vi "Read.vi"(8 "error in (no error)":errorcluster, 11 "Configuration Filename":path) -> (0 "error out":errorcluster, 1 "All items found?":bool, 2 "HGF_Configuration out":refnum<class "HGF_Configuration.lvclass">, 3 "HGF_Application out":refnum<class "HGF_Application.lvclass">)   [LabVIEW 2012, in "HGF_ApplicationBaseClasses.lvlib" / "HGF_Configuration.lvclass"]
uses:
  HGF_Configuration.lvclass
  HGF_Application/HGF_Application.lvclass
  HGF_DesignPatterns/Apps/MyApp/MyAppFactory/MyAppFactory.lvclass
  HGF_Configuration.lvclass/HGF_Configuration.ctl
  <vilib>/Utility/config.llb/Read Key (String).vi
  <vilib>/Utility/config.llb/NI_LVConfig.lvlib
  HGF_BaseClasses/HGF_Factory/HGF_Factory.lvclass
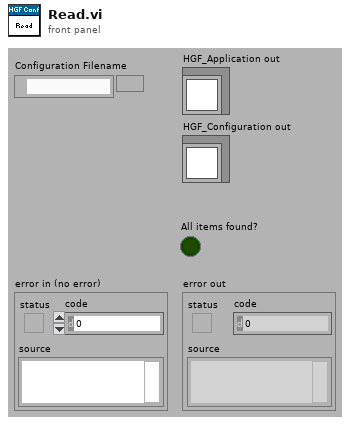
[diagram p1: front panel]
types:
  T1 = typedef "NI_LVConfig.lvlib/Config Data RefNum.ctl" = refnum<k1>
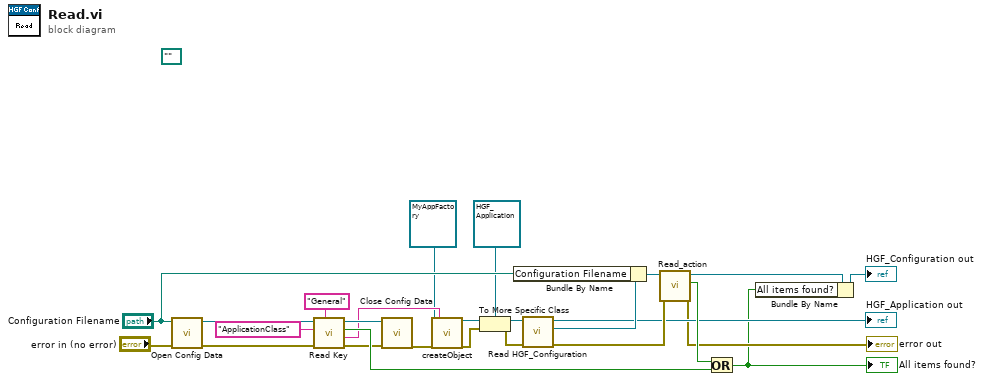
[diagram p0: block diagram]
diagram:
  (unwired) path "" ("Configuration Filename")
  n1 = call <vilib>:"Open Config Data.vi"("error in (no error)"="error in (no error)", "configuration file path"="Configuration Filename") -> ("error out"=w24:errorcluster, "refnum"=w25:T1)  [unwired: 7 in, 1 out]
  n2 = call-poly <vilib>:"Read Key.vi"("section"="General", "error in (no error)"=w24, "key"="ApplicationClass", "refnum"=w25) -> ("error out"=w17:errorcluster, "value"=w16:string, "found?"=w20:bool, "refnum out"=w18:T1)  [unwired: 4 in]
  n3 = call <vilib>:"Close Config Data.vi"("error in (no error)"=w17, "refnum"=w18) -> ("error out"=w8:errorcluster)  [unwired: 8 in, 1 out]
  n4 = call "createObject.vi"("HGF_Factory"=refnum<class "MyAppFactory.lvclass"> refnum ("MyApp.lvlib:MyAppFactory.lvclass"), "error in (no error)"=w8, "className"=w16) -> ("HGF_Object"=w14:refnum<class "HGF_Factory.lvclass">, "error out"=w15:errorcluster)  [unwired: 14 in, 1 out]
  n5 = To More Specific Class(target class=refnum<class "HGF_Application.lvclass"> refnum ("HGF_ApplicationBaseClasses.lvlib:HGF_Application.lvclass"), reference=w14, error in=w15) -> (specific class reference=w11:refnum<class "HGF_Application.lvclass">, error out=w10:errorcluster)
  n6 = call "Read HGF_Configuration.vi"("error in (no error)"=w10, "HGF_Application in"=w11) -> ("error out"=w7:errorcluster, "HGF_Configuration"=w9:refnum<class "HGF_Configuration.lvclass">, "HGF_Application out"=→"HGF_Application out":refnum<class "HGF_Application.lvclass">)  [unwired: 7 in]
  n7 = Bundle By Name(cluster=w9, "Configuration Filename"="Configuration Filename") -> (w13:refnum<class "HGF_Configuration.lvclass">)
  n8 = call-dynamic "Read_action.vi"("error in (no error)"=w7, "HGF_Configuration in"=w13) -> ("error out"=→"error out":errorcluster, "All items found?"=w19:bool, "HGF_Configuration out"=w4:refnum<class "HGF_Configuration.lvclass">)  [unwired: 7 in]
  n9 = Or(x=w19, y=w20) -> (x .or. y?=w2:bool)
  "All items found?" <- w2
  n10 = Bundle By Name(cluster=w4, "All items found?"=w2) -> (→"HGF_Configuration out":refnum<class "HGF_Configuration.lvclass">)
